vi "hse-application_GetGlobalShutdownEvent.vi"(8 "error in":errorcluster) -> (0 "error out":errorcluster, 3 "global shutdown event":refnum<user-event>)   [LabVIEW 2020, in "hse-application.lvclass"]
doc: "Returns information on the application itself for display, logging, ...\n\n\n\n____\nHAMPEL SOFTWARE ENGINEERING v3.8.0 (2023-12-18 14:41)"
uses:
  hse-application.lvclass
  hse-application.lvclass/hse-application.ctl
  <vilib>/Utility/error.llb/Error Cluster From Error Code.vi
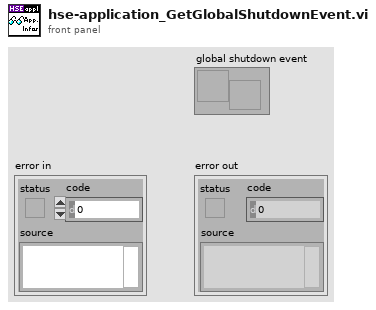
[diagram p1: front panel]
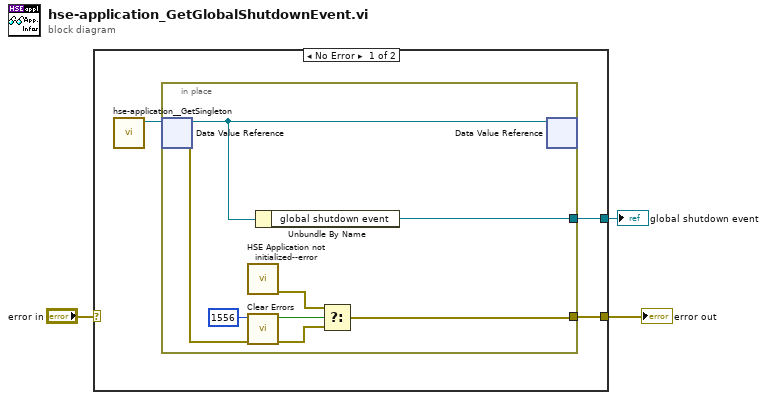
[diagram p0: block diagram]
diagram:
  n1 = case shown="No Error" "error in" {
    selector: "error in" -> [_ w15]
    tunnel: [w6 w15] -> w2
    tunnel: [w4 _] -> w1
    frame No Error {
      n2 = call "hse-application__GetSingleton.vi"() -> ("ApplicationClass DVR"=w5:refnum<data-value>)  [unwired: 10 in, 1 out]
      n3 = in-place {
        in-place-border: [w11] -> w6
        in-place-border: [w9] -> w4
        n4 = in-place-dvr #1(w5) -> (w10:refnum<class "hse-application.lvclass">, w12:errorcluster)
        n5 = call "HSE Application not initialized--error.vi"() -> ("error out"=w14:errorcluster)  [unwired: 11 in]
        n6 = call <vilib>:"Clear Errors.vi"("error in (no error)"=w12, "specific error code to clear (0: all)"=1556) -> ("error out"=w13:errorcluster, "specific error cleared?"=w7:bool)  [unwired: 4 in]
        n7 = Unbundle By Name(w10) -> ("global shutdown event"=w9:refnum<user-event>)
        n8 = Select(t=w14, s=w7, f=w13) -> (s? t:f=w11:errorcluster)
        n9 = in-place-dvr #1(w10) -> ()  [unwired: 2 out]
      }
    }
    frame Error {
    }
  }
  "error out" <- w2
  "global shutdown event" <- w1
